vi "PH_BL-Master.ProcCases.vi"(0 "i ref in":refnum<vi>, 1 "selector":string, 2 "Data":T1, 3 "call cluster":T2={"Object"="", "Selector"="", "CallType"=enum."synchronous", "Async Object"="", "Async Selector"="", "Data Descriptor"="", "Data"=[], "Error #"=0, "Expire"=0}, 5 "error in (no error)":errorcluster) -> (14 "i ref out":refnum<vi>, 17 "answer cluster":T2={"Object"="", "Selector"="", "CallType"=enum."synchronous", "Async Object"="", "Async Selector"="", "Data Descriptor"="", "Data"=[], "Error #"=0, "Expire"=0}, 19 "error out":errorcluster)   [LabVIEW 2014, in "PH_BL-Master.lvlib"]
doc: "This method is called by a process from within the default case in the event loop. The methods of a class that are linked to events will be called from THIS method. Add your code here."
uses:
  PH_BL-Master.lvlib
  CSCore/CSSystem/CoreDefs/CoreDefs.call_type.ctl
  CSCore/BaseProcess/BaseProcess.descriptor string definition.ctl
  CSCore/CSSystem/CoreDefs/CoreDefs.rawDataType.ctl
  CSCore/CSSystem/CSSystemLib/CSSystemLib.object condition.ctl
  PH_BL-Master.Shutter State.ctl
  CSCore/CSSystem/CoreLib/CoreLib.byte array 2 short.vi
  CSCore/CSSystem/CoreLib/CoreLib.string 2 byte array.vi
  CSCore/CSSystem/CoreLib/CoreLib.lvlib
  CSCore/BaseProcess/BaseProcess.lvlib
  CSCore/CAEObj/CAEObj.lvlib
  PH_Common/PH_Common.lvlib
  PH_StatusHandler/PH_StatusHandler.lvlib
  CSCore/CSSystem/CSSystemLib/CSSystemLib.lvlib
  PH_SystemInformation/PH_SystemInformation.lvlib
  PH_4_Pos_Selector/PH_4_Pos_Selector.lvlib
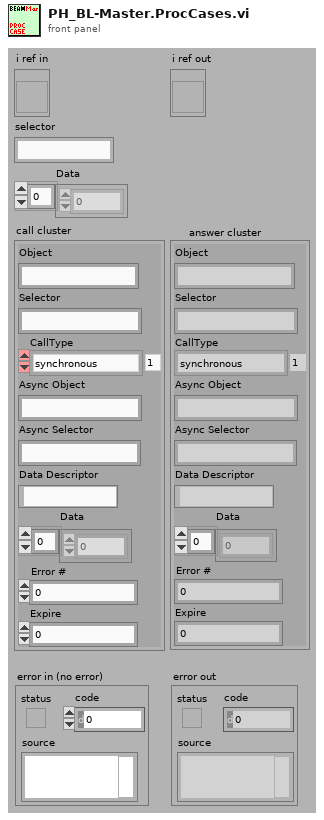
[diagram p1: front panel]
types:
  T1 = typedef "CoreDefs.rawDataType.ctl" = i8[]
  T2 = typedef "CoreDefs.call_type.ctl" = cluster{"Object":string, "Selector":string, "CallType":enum16{"simple", "synchronous", "asynchronous"}, "Async Object":string, "Async Selector":string, "Data Descriptor":T3, "Data":T1, "Error #":i32, "Expire":u32}
  T3 = typedef "BaseProcess.lvlib/BaseProcess.descriptor string definition.ctl" = string
  T4 = typedef "PH_BL-Master.lvlib/PH_BL-Master.Shutter State.ctl" = enum16{"No Link", "No Info", "In", "Out", "in between"}
  T5 = typedef "PH_4_Pos_Selector.lvlib/PH_4_Pos_Selector.Position Selector.ctl" = u16
  T6 = typedef "CSSystemLib.lvlib/CSSystemLib.object condition.ctl" = i32
  T7 = typedef "PH_BL-Master.lvlib/PH_BL-Master.i attribute.ctl" = cluster{"Remote controlled":bool, "Boolean Condition Service Subscriber":refnum<vi>[], "Picture Condition Service Subscriber":refnum<vi>[], "R2S":cluster{"GUI Ref":refnum<vi>, "State":bool}, "Vacua":cluster{"GUI Ref":refnum<vi>, "Limit":dbl, "Curr Value":dbl, "in range":bool}[], "O2 Inspection":cluster{"GUI Ref":refnum<vi>, "Concentration":dbl, "State":T8}[], "Boolean Status Service Subscriber":cluster{"GUI Ref":refnum<vi>, "Status":T8, "no Link?":bool, "Status Subscriber Class":T9}[], "Picture Status Service Subscriber":cluster{"GUI Ref":refnum<vi>, "Status":T8, "no Link?":bool, "Status Subscriber Class":T9}[], "6P 4Q Service Subscriber":cluster{"GUI Ref":refnum<vi>, "Selector":T5, "no Link?":bool}[], "Index of latest 6P 4Q changing Instance":i32, "Index of latest Picture Status changing Instance":i32, "Index of latest Boolean Status changing Instance":i32, "Vision ID on same Node":string, "Start Phase over?":bool, "GUI Ref Delete":refnum<vi>}
  T8 = typedef "PH_StatusHandler.lvlib/PH_StatusHandler.Status.ctl" = i16
  T9 = typedef "PH_BL-Master.lvlib/PH_BL-Master.Status Subscriber Class.ctl" = enum16{"unknown", "Switch", "BB", "6P Switch", "Switch GUI", "Switch and 6P State", "Force Sensor"}
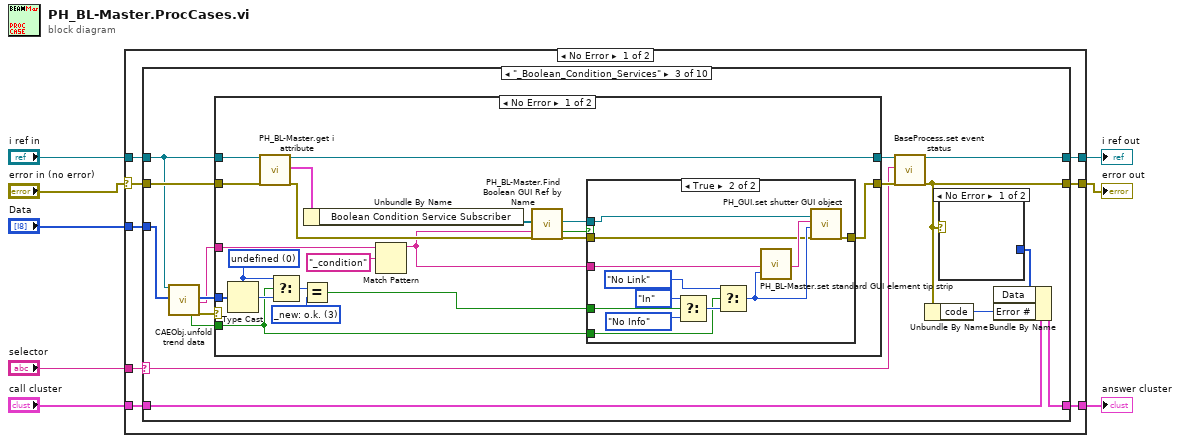
[diagram p0: block diagram]
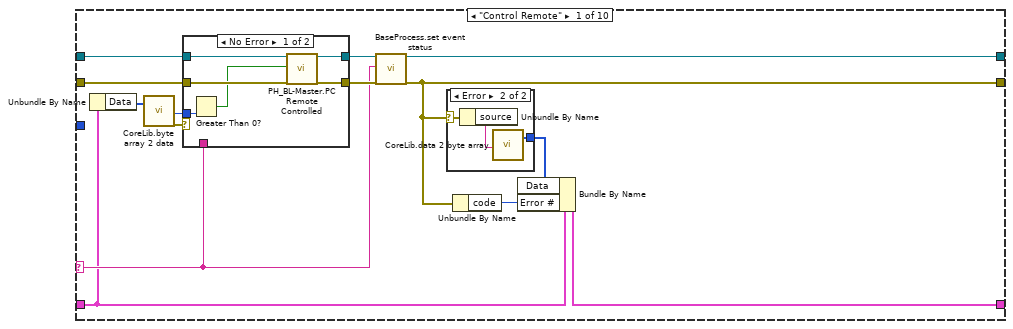
[diagram p2: hidden frame]
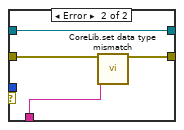
[diagram p4: hidden frame]
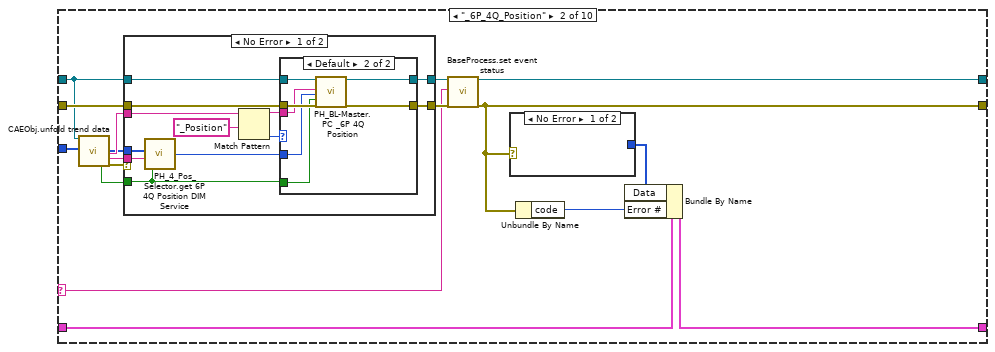
[diagram p5: hidden frame]
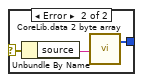
[diagram p6: hidden frame]
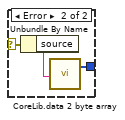
[diagram p9: hidden frame]
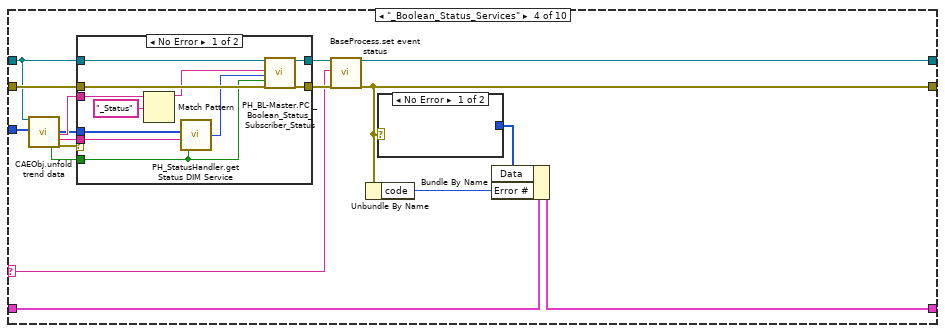
[diagram p12: hidden frame]
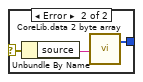
[diagram p13: hidden frame]
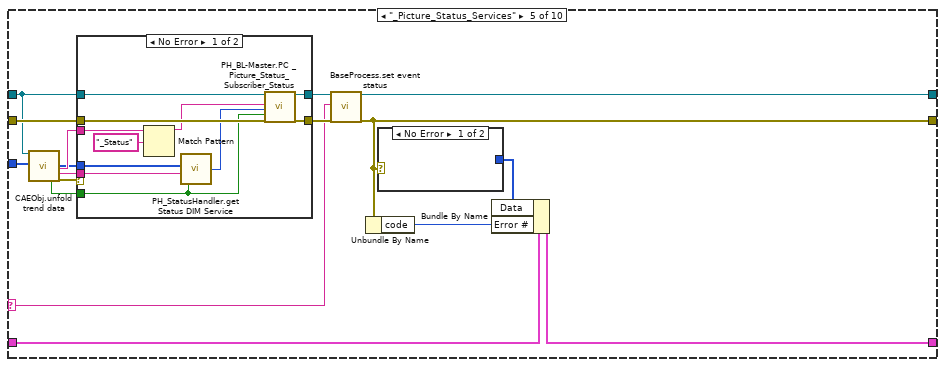
[diagram p15: hidden frame]
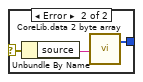
[diagram p16: hidden frame]
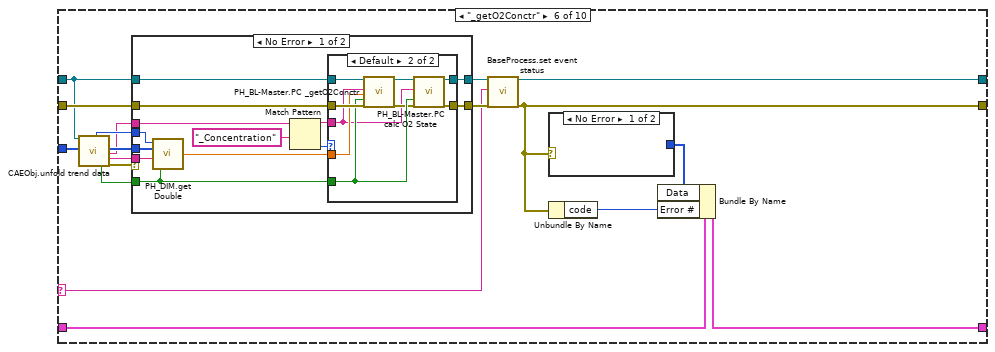
[diagram p18: hidden frame]
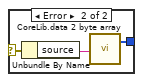
[diagram p19: hidden frame]
diagram:
  n1 = case shown="No Error" "error in (no error)" {
    selector: "error in (no error)" -> [w9 w401]
    tunnel: "selector" -> [w16 _]
    tunnel: [w15 w400] -> w7
    tunnel: "call cluster" -> [w14 w400]
    tunnel: "i ref in" -> [w13 w402]
    tunnel: [w12 w402] -> w4
    tunnel: [w11 w401] -> w3
    tunnel: "Data" -> [w10 _]
    frame No Error {
      n2 = case shown="\"_Boolean_Condition_Services\"" w16 {
        selector: w16 -> [w19 w48 w90 w145 w178 w209 w256 w304 w351 w397]
        tunnel: w13 -> [w30 w58 w100 w155 w188 w222 w269 w317 w361 w395]
        tunnel: [w21 w50 w92 w144 w177 w211 w258 w307 w353 w393] -> w12
        tunnel: w14 -> [w18 w47 w89 w142 w175 w208 w255 w305 w350 w398]
        tunnel: [w17 w46 w88 w141 w174 w207 w254 w303 w349 w399] -> w15
        tunnel: w9 -> [w29 w60 w102 w157 w190 w224 w271 w320 w363 w394]
        tunnel: [w20 w49 w91 w143 w176 w210 w257 w306 w352 w392] -> w11
        tunnel: w10 -> [_ w59 w101 w156 w189 w223 w270 w319 w362 w396]
        frame "Control Remote" {
          n3 = Unbundle By Name(w18) -> ("Data"=w28:T1)
          n4 = call-poly "CoreLib.byte array 2 data.vi"("byteArray"=w28) -> ("i16"=w27:i16, "error out"=w26:errorcluster)  [unwired: 16 in, 1 out]
          n5 = case shown="No Error" w26 {
            tunnel: [w37 w43] -> w23
            tunnel: w30 -> [w38 w43]
            tunnel: w29 -> [w39 w42]
            tunnel: [w36 w41] -> w22
            tunnel: w19 -> [_ w40]
            tunnel: w27 -> [w35 _]
            frame No Error {
              n6 = Greater Than 0?(x=w35) -> (x > 0?=w34:bool)
              n7 = call "PH_BL-Master.PC Remote Controlled.vi"("i ref in"=w38, "Remote controlled"=w34, "error in (no error)"=w39) -> ("i ref out"=w37:refnum<vi>, "error out"=w36:errorcluster)  [unwired: 15 in]
            }
            frame Error {
              n8 = call "CoreLib.set data type mismatch.vi"("error in (no error)"=w42, "error source"=w40) -> ("error out"=w41:errorcluster)  [unwired: 17 in]
            }
          }
          n9 = call "BaseProcess.set event status.vi"("i ref in"=w23, "EventStatus"=w19, "error in (no error)"=w22) -> ("i ref out"=w21:refnum<vi>, "error out"=w20:errorcluster)  [unwired: 14 in, 1 out]
          n10 = case shown="Error" w20 {
            selector: w20 -> [_ w33]
            tunnel: [_ w31] -> w24
            frame No Error {
            }
            frame Error {
              n11 = Unbundle By Name(w33) -> ("source"=w32:string)
              n12 = call-poly "CoreLib.data 2 byte array.vi"("string"=w32) -> ("byteArray out"=w31:T1)  [unwired: 18 in]
            }
          }
          n13 = Unbundle By Name(w20) -> ("code"=w25:i32)
          n14 = Bundle By Name(cluster=w18, "Data"=w24, "Error #"=w25) -> (w17:T2)
        }
        frame "_6P_4Q_Position" {
          n15 = call "CAEObj.unfold trend data.vi"("i ref in"=w58, "raw trend data"=w59) -> ("no link"=w56:bool, "data"=w44:i8[], "serviceName"=w55:string, "typeDescriptor"=w45:string, "error out"=w57:errorcluster)  [unwired: 9 in, 4 out]
          n16 = case shown="No Error" w57 {
            tunnel: [w69 w86] -> w52
            tunnel: w58 -> [w74 w86]
            tunnel: w60 -> [w75 w85]
            tunnel: [w68 w85] -> w51
            tunnel: w56 -> [w72 _]
            tunnel: w55 -> [w66 _]
            tunnel: w45 -> [w71 _]
            tunnel: w44 -> [w70 _]
            frame No Error {
              n17 = call "PH_4_Pos_Selector.get 6P 4Q Position DIM Service.vi"("no link"=w72, "typeDescriptor"=w71, "data"=w70) -> ("Position"=w73:T5)  [unwired: 1 in]
              n18 = Match Pattern(string=w66, regular expression="_Position") -> (before substring=w65:string, offset past match=w64:i32)  [unwired: 1 in, 2 out]
              n19 = case shown="Default" w64 {
                tunnel: w75 -> [w76 w84]
                tunnel: w74 -> [w77 w83]
                tunnel: w73 -> [_ w82]
                tunnel: w72 -> [_ w78]
                tunnel: [w77 w79] -> w69
                tunnel: [w76 w80] -> w68
                tunnel: w65 -> [_ w81]
                frame -1 {
                }
                frame Default {
                  n20 = call "PH_BL-Master.PC _6P 4Q Position.vi"("i ref in"=w83, "6P 4Q Instance"=w81, "Selector"=w82, "no Link"=w78, "error in (no error)"=w84) -> ("i ref out"=w79:refnum<vi>, "error out"=w80:errorcluster)  [unwired: 13 in]
                }
              }
            }
            frame Error {
            }
          }
          n21 = call "BaseProcess.set event status.vi"("i ref in"=w52, "EventStatus"=w48, "error in (no error)"=w51) -> ("i ref out"=w50:refnum<vi>, "error out"=w49:errorcluster)  [unwired: 14 in, 1 out]
          n22 = case shown="No Error" w49 {
            selector: w49 -> [_ w63]
            tunnel: [_ w61] -> w53
            frame No Error {
            }
            frame Error {
              n23 = Unbundle By Name(w63) -> ("source"=w62:string)
              n24 = call-poly "CoreLib.data 2 byte array.vi"("string"=w62) -> ("byteArray out"=w61:T1)  [unwired: 18 in]
            }
          }
          n25 = Unbundle By Name(w49) -> ("code"=w54:i32)
          n26 = Bundle By Name(cluster=w47, "Data"=w53, "Error #"=w54) -> (w46:T2)
        }
        frame "_Boolean_Condition_Services" {
          n27 = call "CAEObj.unfold trend data.vi"("i ref in"=w100, "raw trend data"=w101) -> ("no link"=w97:bool, "data"=w98:i8[], "serviceName"=w87:string, "error out"=w99:errorcluster)  [unwired: 9 in, 5 out]
          n28 = case shown="No Error" w99 {
            tunnel: [w112 w140] -> w94
            tunnel: w100 -> [w123 w140]
            tunnel: w102 -> [w122 w139]
            tunnel: [w113 w139] -> w93
            tunnel: w98 -> [w121 _]
            tunnel: w97 -> [w114 _]
            tunnel: w87 -> [w117 _]
            frame No Error {
              w119 = T6 3 items=["undefined", "executing constructor", "_new: error", "_new: o.k.", "executing destructor"] ("x")
              w124 = T6 0 items=["undefined", "executing constructor", "_new: error", "_new: o.k.", "executing destructor"] ("condition")
              n29 = Type Cast(type=w124, x=w121) -> (*(type *) &x=w125:T6)
              n30 = call "PH_BL-Master.get i attribute.vi"("i ref in"=w123, "error in (no error)"=w122) -> ("i ref out"=w112:refnum<vi>, "i attribute"=w118:T7, "error out"=w111:errorcluster)  [unwired: 15 in]
              n31 = Select(t=w124, s=w114, f=w125) -> (s? t:f=w120:T6)
              n32 = Equal?(x=w120, y=w119) -> (x = y?=w115:bool)
              n33 = Unbundle By Name(w118) -> ("Boolean Condition Service Subscriber"=w106:refnum<vi>[])
              n34 = Match Pattern(string=w117, regular expression="_condition") -> (before substring=w109:string)  [unwired: 1 in, 3 out]
              n35 = call "PH_BL-Master.Find Boolean GUI Ref by Name.vi"("Boolean Ref Array"=w106, "Label"=w109, "error in (no error)"=w111) -> ("Wanted Boolean Ref"=w107:refnum<vi>, "Ref found?"=w108:bool, "error out"=w110:errorcluster)  [unwired: 13 in, 1 out]
              n36 = case shown="True" w108 {
                tunnel: w115 -> [_ w138]
                tunnel: w110 -> [w126 w128]
                tunnel: w114 -> [_ w133]
                tunnel: [w126 w132] -> w113
                tunnel: w107 -> [_ w127]
                tunnel: w109 -> [_ w130]
                frame False {
                }
                frame True {
                  n37 = Select(t=PH_BL-Master.Shutter_State."In", s=w138, f=PH_BL-Master.Shutter_State."No Info" ("Shutter State")) -> (s? t:f=w134:T4)
                  n38 = Select(t=PH_BL-Master.Shutter_State."No Link" ("Shutter State"), s=w133, f=w134) -> (s? t:f=w131:T4)
                  n39 = call "PH_BL-Master.set standard GUI element tip strip.vi"("Instance Name"=w130, "Element State"=w131) -> ("Tip Strip"=w129:string)  [unwired: 17 in]
                  n40 = call "PH_GUI.set shutter GUI object.vi"("Wanted Boolean Ref"=w127, "Tip Strip"=w129, "Shutter State"=w131, "error in (no error)"=w128) -> ("error out"=w132:errorcluster)  [unwired: 15 in]
                }
              }
            }
            frame Error {
            }
          }
          n41 = call "BaseProcess.set event status.vi"("i ref in"=w94, "EventStatus"=w90, "error in (no error)"=w93) -> ("i ref out"=w92:refnum<vi>, "error out"=w91:errorcluster)  [unwired: 14 in, 1 out]
          n42 = Unbundle By Name(w91) -> ("code"=w96:i32)
          n43 = case shown="No Error" w91 {
            selector: w91 -> [_ w105]
            tunnel: [_ w103] -> w95
            frame No Error {
            }
            frame Error {
              n44 = Unbundle By Name(w105) -> ("source"=w104:string)
              n45 = call-poly "CoreLib.data 2 byte array.vi"("string"=w104) -> ("byteArray out"=w103:T1)  [unwired: 18 in]
            }
          }
          n46 = Bundle By Name(cluster=w89, "Data"=w95, "Error #"=w96) -> (w88:T2)
        }
        frame "_Boolean_Status_Services" {
          n47 = call "CAEObj.unfold trend data.vi"("i ref in"=w155, "raw trend data"=w156) -> ("no link"=w151:bool, "data"=w150:i8[], "serviceName"=w153:string, "typeDescriptor"=w152:string, "error out"=w154:errorcluster)  [unwired: 9 in, 4 out]
          n48 = case shown="No Error" w154 {
            tunnel: [w166 w173] -> w147
            tunnel: w155 -> [w170 w173]
            tunnel: w157 -> [w171 w172]
            tunnel: [w165 w172] -> w146
            tunnel: w153 -> [w163 _]
            tunnel: w152 -> [w169 _]
            tunnel: w151 -> [w161 _]
            tunnel: w150 -> [w168 _]
            frame No Error {
              n49 = Match Pattern(string=w163, regular expression="_Status") -> (before substring=w162:string)  [unwired: 1 in, 3 out]
              n50 = call "PH_StatusHandler.get Status DIM Service.vi"("no link"=w161, "typeDescriptor"=w169, "data"=w168) -> ("Status"=w167:T8)  [unwired: 1 in]
              n51 = call "PH_BL-Master.PC _Boolean_Status_Subscriber_Status.vi"("i ref in"=w170, "Boolean Subscriber Instance Name"=w162, "Status"=w167, "no Link?"=w161, "error in (no error)"=w171) -> ("i ref out"=w166:refnum<vi>, "error out"=w165:errorcluster)  [unwired: 13 in]
            }
            frame Error {
            }
          }
          n52 = call "BaseProcess.set event status.vi"("i ref in"=w147, "EventStatus"=w145, "error in (no error)"=w146) -> ("i ref out"=w144:refnum<vi>, "error out"=w143:errorcluster)  [unwired: 14 in, 1 out]
          n53 = Unbundle By Name(w143) -> ("code"=w149:i32)
          n54 = case shown="No Error" w143 {
            selector: w143 -> [_ w160]
            tunnel: [_ w158] -> w148
            frame No Error {
            }
            frame Error {
              n55 = Unbundle By Name(w160) -> ("source"=w159:string)
              n56 = call-poly "CoreLib.data 2 byte array.vi"("string"=w159) -> ("byteArray out"=w158:T1)  [unwired: 18 in]
            }
          }
          n57 = Bundle By Name(cluster=w142, "Data"=w148, "Error #"=w149) -> (w141:T2)
        }
        frame "_Picture_Status_Services" {
          n58 = call "CAEObj.unfold trend data.vi"("i ref in"=w188, "raw trend data"=w189) -> ("no link"=w184:bool, "data"=w183:i8[], "serviceName"=w186:string, "typeDescriptor"=w185:string, "error out"=w187:errorcluster)  [unwired: 9 in, 4 out]
          n59 = case shown="No Error" w187 {
            tunnel: [w199 w206] -> w180
            tunnel: w188 -> [w203 w206]
            tunnel: w190 -> [w204 w205]
            tunnel: [w198 w205] -> w179
            tunnel: w186 -> [w196 _]
            tunnel: w185 -> [w202 _]
            tunnel: w184 -> [w195 _]
            tunnel: w183 -> [w201 _]
            frame No Error {
              n60 = Match Pattern(string=w196, regular expression="_Status") -> (before substring=w194:string)  [unwired: 1 in, 3 out]
              n61 = call "PH_StatusHandler.get Status DIM Service.vi"("no link"=w195, "typeDescriptor"=w202, "data"=w201) -> ("Status"=w200:T8)  [unwired: 1 in]
              n62 = call "PH_BL-Master.PC _Picture_Status_Subscriber_Status.vi"("i ref in"=w203, "Picture Subscriber Instance Name"=w194, "Status"=w200, "no Link?"=w195, "error in (no error)"=w204) -> ("i ref out"=w199:refnum<vi>, "error out"=w198:errorcluster)  [unwired: 13 in]
            }
            frame Error {
            }
          }
          n63 = call "BaseProcess.set event status.vi"("i ref in"=w180, "EventStatus"=w178, "error in (no error)"=w179) -> ("i ref out"=w177:refnum<vi>, "error out"=w176:errorcluster)  [unwired: 14 in, 1 out]
          n64 = Unbundle By Name(w176) -> ("code"=w182:i32)
          n65 = case shown="No Error" w176 {
            selector: w176 -> [_ w193]
            tunnel: [_ w191] -> w181
            frame No Error {
            }
            frame Error {
              n66 = Unbundle By Name(w193) -> ("source"=w192:string)
              n67 = call-poly "CoreLib.data 2 byte array.vi"("string"=w192) -> ("byteArray out"=w191:T1)  [unwired: 18 in]
            }
          }
          n68 = Bundle By Name(cluster=w175, "Data"=w181, "Error #"=w182) -> (w174:T2)
        }
        frame "_getO2Conctr" {
          n69 = call "CAEObj.unfold trend data.vi"("i ref in"=w222, "raw trend data"=w223) -> ("quality"=w218:i32, "no link"=w217:bool, "data"=w219:i8[], "serviceName"=w216:string, "typeDescriptor"=w220:string, "error out"=w221:errorcluster)  [unwired: 9 in, 3 out]
          n70 = case shown="No Error" w221 {
            tunnel: [w233 w253] -> w213
            tunnel: w222 -> [w239 w253]
            tunnel: w224 -> [w240 w252]
            tunnel: [w232 w252] -> w212
            tunnel: w220 -> [w238 _]
            tunnel: w219 -> [w237 _]
            tunnel: w218 -> [w236 _]
            tunnel: w217 -> [w234 _]
            tunnel: w216 -> [w230 _]
            frame No Error {
              n71 = call "PH_DIM.get Double.vi"("no link"=w234, "typeDescriptor"=w238, "data"=w237, "quality"=w236) -> ("Value"=w235:dbl)
              n72 = Match Pattern(string=w230, regular expression="_Concentration") -> (before substring=w229:string, offset past match=w228:i32)  [unwired: 1 in, 2 out]
              n73 = case shown="Default" w228 {
                tunnel: w240 -> [w241 w251]
                tunnel: w239 -> [w242 w250]
                tunnel: w235 -> [_ w249]
                tunnel: w234 -> [_ w248]
                tunnel: [w242 w245] -> w233
                tunnel: [w241 w244] -> w232
                tunnel: w229 -> [_ w243]
                frame -1 {
                }
                frame Default {
                  n74 = call "PH_BL-Master.PC _getO2Conctr.vi"("i ref in"=w250, "O2 Instance"=w243, "Concentration [%]"=w249, "no link"=w248, "error in (no error)"=w251) -> ("i ref out"=w246:refnum<vi>, "error out"=w247:errorcluster)  [unwired: 13 in]
                  n75 = call "PH_BL-Master.PC calc O2 State.vi"("i ref in"=w246, "O2 Instance"=w243, "no link"=w248, "error in (no error)"=w247) -> ("i ref out"=w245:refnum<vi>, "error out"=w244:errorcluster)  [unwired: 14 in]
                }
              }
            }
            frame Error {
            }
          }
          n76 = call "BaseProcess.set event status.vi"("i ref in"=w213, "EventStatus"=w209, "error in (no error)"=w212) -> ("i ref out"=w211:refnum<vi>, "error out"=w210:errorcluster)  [unwired: 14 in, 1 out]
          n77 = case shown="No Error" w210 {
            selector: w210 -> [_ w227]
            tunnel: [_ w225] -> w214
            frame No Error {
            }
            frame Error {
              n78 = Unbundle By Name(w227) -> ("source"=w226:string)
              n79 = call-poly "CoreLib.data 2 byte array.vi"("string"=w226) -> ("byteArray out"=w225:T1)  [unwired: 18 in]
            }
          }
          n80 = Unbundle By Name(w210) -> ("code"=w215:i32)
          n81 = Bundle By Name(cluster=w208, "Data"=w214, "Error #"=w215) -> (w207:T2)
        }
        frame "_getVacLimits" {
          n82 = call "CAEObj.unfold trend data.vi"("i ref in"=w269, "raw trend data"=w270) -> ("quality"=w265:i32, "no link"=w264:bool, "data"=w266:i8[], "serviceName"=w263:string, "typeDescriptor"=w267:string, "error out"=w268:errorcluster)  [unwired: 9 in, 3 out]
          n83 = case shown="No Error" w268 {
            tunnel: [w280 w302] -> w260
            tunnel: w269 -> [w286 w302]
            tunnel: w271 -> [w287 w301]
            tunnel: [w279 w301] -> w259
            tunnel: w267 -> [w285 _]
            tunnel: w266 -> [w284 _]
            tunnel: w265 -> [w283 _]
            tunnel: w264 -> [w281 _]
            tunnel: w263 -> [w278 _]
            frame No Error {
              n84 = call "PH_DIM.get Double.vi"("no link"=w281, "typeDescriptor"=w285, "data"=w284, "quality"=w283) -> ("Value"=w282:dbl)
              n85 = Match Pattern(string=w278, regular expression="_Limit") -> (before substring=w276:string, offset past match=w275:i32)  [unwired: 1 in, 2 out]
              n86 = case shown="Default" w275 {
                tunnel: w287 -> [w288 w300]
                tunnel: w286 -> [w289 w299]
                tunnel: w282 -> [_ w298]
                tunnel: w281 -> [_ w295]
                tunnel: [w289 w294] -> w280
                tunnel: [w288 w293] -> w279
                tunnel: w276 -> [_ w290]
                frame -1 {
                }
                frame Default {
                  n87 = call "PH_BL-Master.PC _getVacLimits.vi"("i ref in"=w299, "Channelname"=w290, "Value"=w298, "no link"=w295, "error in (no error)"=w300) -> ("i ref out"=w297:refnum<vi>, "error out"=w296:errorcluster)  [unwired: 13 in]
                  n88 = call "PH_BL-Master.PC calc Vac State.vi"("i ref in"=w297, "Channel Name"=w290, "no link"=w295, "error in (no error)"=w296) -> ("i ref out"=w292:refnum<vi>, "error out"=w291:errorcluster)  [unwired: 14 in]
                  n89 = call "PH_BL-Master.set vacuum Gui element tip strips.vi"("i ref in"=w292, "error in (no error)"=w291) -> ("i ref out"=w294:refnum<vi>, "error out"=w293:errorcluster)  [unwired: 16 in]
                }
              }
            }
            frame Error {
            }
          }
          n90 = call "BaseProcess.set event status.vi"("i ref in"=w260, "EventStatus"=w256, "error in (no error)"=w259) -> ("i ref out"=w258:refnum<vi>, "error out"=w257:errorcluster)  [unwired: 14 in, 1 out]
          n91 = case shown="No Error" w257 {
            selector: w257 -> [_ w274]
            tunnel: [_ w272] -> w261
            frame No Error {
            }
            frame Error {
              n92 = Unbundle By Name(w274) -> ("source"=w273:string)
              n93 = call-poly "CoreLib.data 2 byte array.vi"("string"=w273) -> ("byteArray out"=w272:T1)  [unwired: 18 in]
            }
          }
          n94 = Unbundle By Name(w257) -> ("code"=w262:i32)
          n95 = Bundle By Name(cluster=w255, "Data"=w261, "Error #"=w262) -> (w254:T2)
        }
        frame "_getVacPressures" {
          n96 = call "CAEObj.unfold trend data.vi"("i ref in"=w317, "raw trend data"=w319) -> ("quality"=w316:i32, "no link"=w313:bool, "data"=w315:i8[], "serviceName"=w312:string, "typeDescriptor"=w314:string, "error out"=w318:errorcluster)  [unwired: 9 in, 3 out]
          n97 = case shown="No Error" w318 {
            tunnel: [w329 w346] -> w309
            tunnel: w317 -> [w335 w346]
            tunnel: w320 -> [w336 w345]
            tunnel: [w328 w345] -> w308
            tunnel: w316 -> [w334 _]
            tunnel: w315 -> [w333 _]
            tunnel: w314 -> [w332 _]
            tunnel: w313 -> [w330 _]
            tunnel: w312 -> [w327 _]
            frame No Error {
              n98 = call "PH_DIM.get Double.vi"("no link"=w330, "typeDescriptor"=w332, "data"=w333, "quality"=w334) -> ("Value"=w331:dbl)
              n99 = Match Pattern(string=w327, regular expression="_Pressure") -> (before substring=w326:string, offset past match=w324:i32)  [unwired: 1 in, 2 out]
              n100 = case shown="Default" w324 {
                tunnel: w336 -> [w337 w344]
                tunnel: w335 -> [w338 w343]
                tunnel: w331 -> [_ w342]
                tunnel: [w338 w341] -> w329
                tunnel: [w337 w340] -> w328
                tunnel: w326 -> [_ w339]
                frame -1 {
                }
                frame Default {
                  n101 = call "PH_BL-Master.PC _getVacPressuress.vi"("i ref in"=w343, "Channel Name"=w339, "Value"=w342, "error in (no error)"=w344) -> ("i ref out"=w341:refnum<vi>, "error out"=w340:errorcluster)  [unwired: 14 in]
                }
              }
            }
            frame Error {
            }
          }
          n102 = call "BaseProcess.set event status.vi"("i ref in"=w309, "EventStatus"=w304, "error in (no error)"=w308) -> ("i ref out"=w307:refnum<vi>, "error out"=w306:errorcluster)  [unwired: 14 in, 1 out]
          n103 = case shown="No Error" w306 {
            selector: w306 -> [_ w323]
            tunnel: [_ w321] -> w310
            frame No Error {
            }
            frame Error {
              n104 = Unbundle By Name(w323) -> ("source"=w322:string)
              n105 = call-poly "CoreLib.data 2 byte array.vi"("string"=w322) -> ("byteArray out"=w321:T1)  [unwired: 18 in]
            }
          }
          n106 = Unbundle By Name(w306) -> ("code"=w311:i32)
          n107 = Bundle By Name(cluster=w305, "Data"=w310, "Error #"=w311) -> (w303:T2)
        }
        frame "_linkO2Conctr" {
          n108 = call "CAEObj.unfold trend data.vi"("i ref in"=w361, "raw trend data"=w362) -> ("no link"=w359:bool, "data"=w347:i8[], "serviceName"=w358:string, "typeDescriptor"=w348:string, "error out"=w360:errorcluster)  [unwired: 9 in, 4 out]
          n109 = case shown="No Error" w360 {
            tunnel: [w372 w391] -> w355
            tunnel: w361 -> [w377 w391]
            tunnel: w363 -> [w378 w390]
            tunnel: [w371 w390] -> w354
            tunnel: w359 -> [w375 _]
            tunnel: w358 -> [w369 _]
            tunnel: w348 -> [w374 _]
            tunnel: w347 -> [w373 _]
            frame No Error {
              n110 = call "PH_StatusHandler.get Status DIM Service.vi"("no link"=w375, "typeDescriptor"=w374, "data"=w373) -> ("Status"=w376:T8)  [unwired: 1 in]
              n111 = Match Pattern(string=w369, regular expression="_Status") -> (before substring=w368:string, offset past match=w367:i32)  [unwired: 1 in, 2 out]
              n112 = case shown="Default" w367 {
                tunnel: w378 -> [w379 w389]
                tunnel: w377 -> [w380 w388]
                tunnel: w376 -> [_ w387]
                tunnel: w375 -> [_ w386]
                tunnel: [w380 w383] -> w372
                tunnel: [w379 w382] -> w371
                tunnel: w368 -> [_ w381]
                frame -1 {
                }
                frame Default {
                  n113 = call "PH_BL-Master.PC _getO2DevStatus.vi"("i ref in"=w388, "O2 Instance"=w381, "Status"=w387, "error in (no error)"=w389) -> ("i ref out"=w384:refnum<vi>, "error out"=w385:errorcluster)  [unwired: 14 in]
                  n114 = call "PH_BL-Master.PC calc O2 State.vi"("i ref in"=w384, "O2 Instance"=w381, "no link"=w386, "error in (no error)"=w385) -> ("i ref out"=w383:refnum<vi>, "error out"=w382:errorcluster)  [unwired: 14 in]
                }
              }
            }
            frame Error {
            }
          }
          n115 = call "BaseProcess.set event status.vi"("i ref in"=w355, "EventStatus"=w351, "error in (no error)"=w354) -> ("i ref out"=w353:refnum<vi>, "error out"=w352:errorcluster)  [unwired: 14 in, 1 out]
          n116 = case shown="No Error" w352 {
            selector: w352 -> [_ w366]
            tunnel: [_ w364] -> w356
            frame No Error {
            }
            frame Error {
              n117 = Unbundle By Name(w366) -> ("source"=w365:string)
              n118 = call-poly "CoreLib.data 2 byte array.vi"("string"=w365) -> ("byteArray out"=w364:T1)  [unwired: 18 in]
            }
          }
          n119 = Unbundle By Name(w352) -> ("code"=w357:i32)
          n120 = Bundle By Name(cluster=w350, "Data"=w356, "Error #"=w357) -> (w349:T2)
        }
        frame Default {
          n121 = call "PH_SystemInformation.ProcCases.vi"("i ref in"=w395, "selector"=w397, "Data"=w396, "call cluster"=w398, "error in (no error)"=w394) -> ("i ref out"=w393:refnum<vi>, "answer cluster"=w399:T2, "error out"=w392:errorcluster)  [unwired: 12 in]
        }
      }
    }
    frame Error {
    }
  }
  "answer cluster" <- w7
  "i ref out" <- w4
  "error out" <- w3
